vi "Serial_CommModule.vi"(8 "error in (no error)":errorcluster) -> (0 "error out":errorcluster)   [LabVIEW 2021]
uses:
  QueueEnum.ctl
  TCPCommModuleData.ctl
  TCPQueueData.ctl
  TCPModuleState.ctl
  ModelQueueCluster.ctl
  ToModelSourceEnum.ctl
  FromTCPCluster.ctl
  ToModelFromTCPMessage.ctl
  FormControllerToMOdelCluster.ctl
  ToModelFromControllerEnum.ctl
  ToSerialCommand.ctl
  ToSerialCTL.ctl
  <vilib>/Instr/_visa.llb/VISA Open Access Mode.ctl
  <vilib>/Instr/_visa.llb/VISA Configure Serial Port (Instr).vi
panel:
  out "bytes written":i32
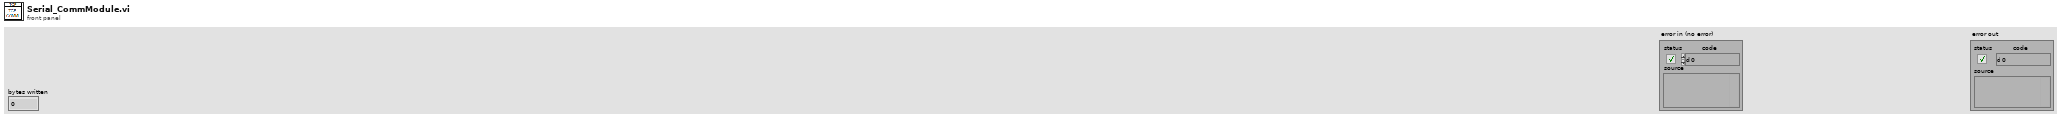
[diagram p1: front panel]
types:
  T1 = typedef "ToSerialCTL.ctl" = enum16{"Init", "Write", "Close", "Read", "Disconnect", "Connect", "Exit", "Error_Handler"}
  T2 = typedef "TCPCommModuleData.ctl" = cluster{"TCP Connection ID":refnum<k5>, "ToTCPModuleQueue":refnum<queue>, "ToModelQueue":refnum<queue>, "Timeout count":u32, "Connected OK?":bool, "ToSerialQueue":refnum<queue>, "VISA resource name":refnum<visa-resource-name>}
  T3 = typedef "QueueEnum.ctl" = enum16{"Obtain Queue", "Get Queue Ref", "Flush Queue", "Release Queue"}
  T4 = enum32{"Invalid", "Standard", "Closed", "Hidden", "Minimized", "Maximized"}
  T5 = typedef "ToSerialCommand.ctl" = cluster{"Command":T1, "VISA resource name":refnum<visa-resource-name>, "Data":string}
  T6 = typedef "ModelQueueCluster.ctl" = cluster{"Source":T7, "FromCommunication":T8, "FromControllerCluster":T10}
  T7 = typedef "ToModelSourceEnum.ctl" = enum16{"COM", "TCP", "Controller"}
  T8 = typedef "FromTCPCluster.ctl" = cluster{"Message":T9, "Data":string, "StatusOK?":bool}
  T9 = typedef "ToModelFromTCPMessage.ctl" = enum16{"Exit", "DataWritten", "DataReceived", "Timeout", "UnableToConnect", "Disconnected", "Connected"}
  T10 = typedef "FormControllerToMOdelCluster.ctl" = cluster{"Command":T11, "IP Address":string, "Remote Port":u16, "Data":string, "TCP/COM":bool, "VISA resource name":refnum<visa-resource-name>}
  T11 = typedef "ToModelFromControllerEnum.ctl" = enum16{"StopLogging", "StartLogging", "SlideChange", "SendMessage", "Exit", "Disconnect", "Connect"}
  T12 = typedef "VISA Open Access Mode.ctl" = u32
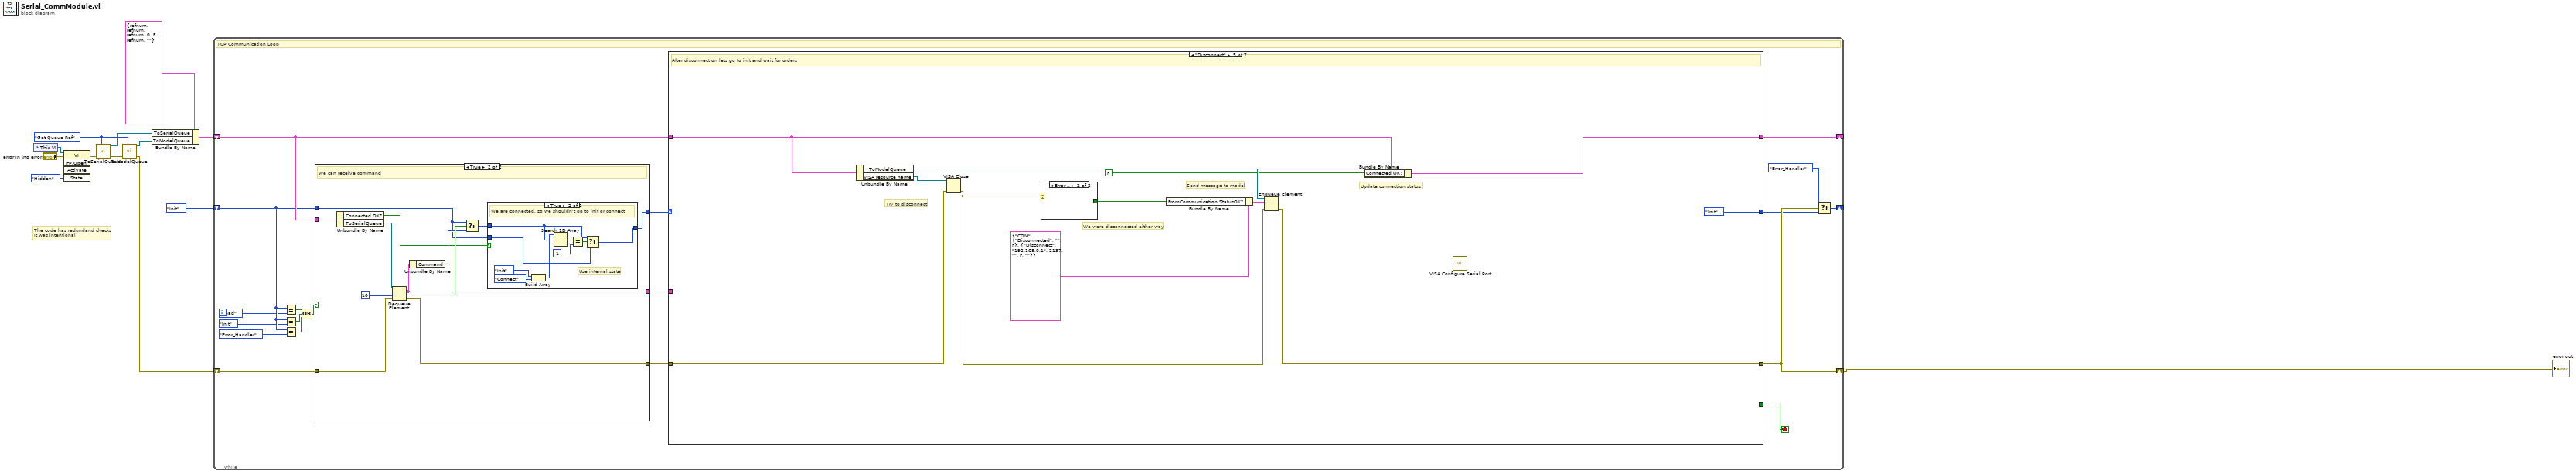
[diagram p0: block diagram]
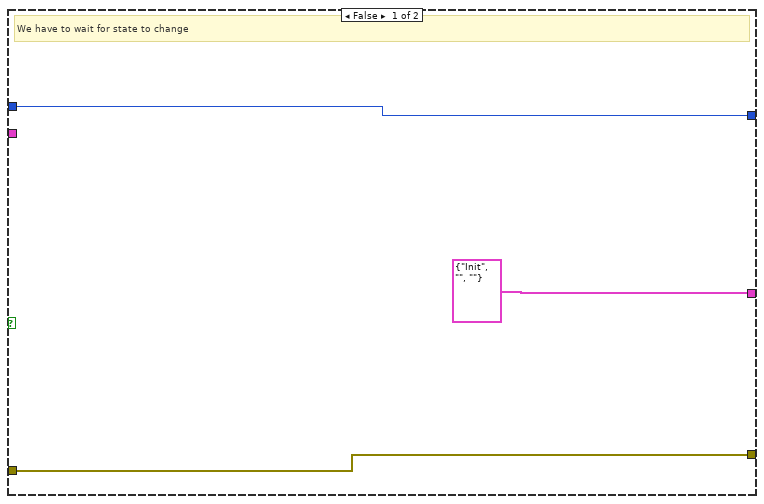
[diagram p2: hidden frame]
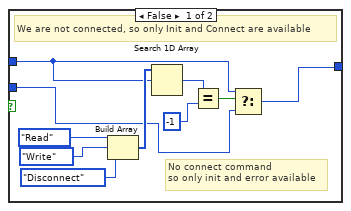
[diagram p3: hidden frame]
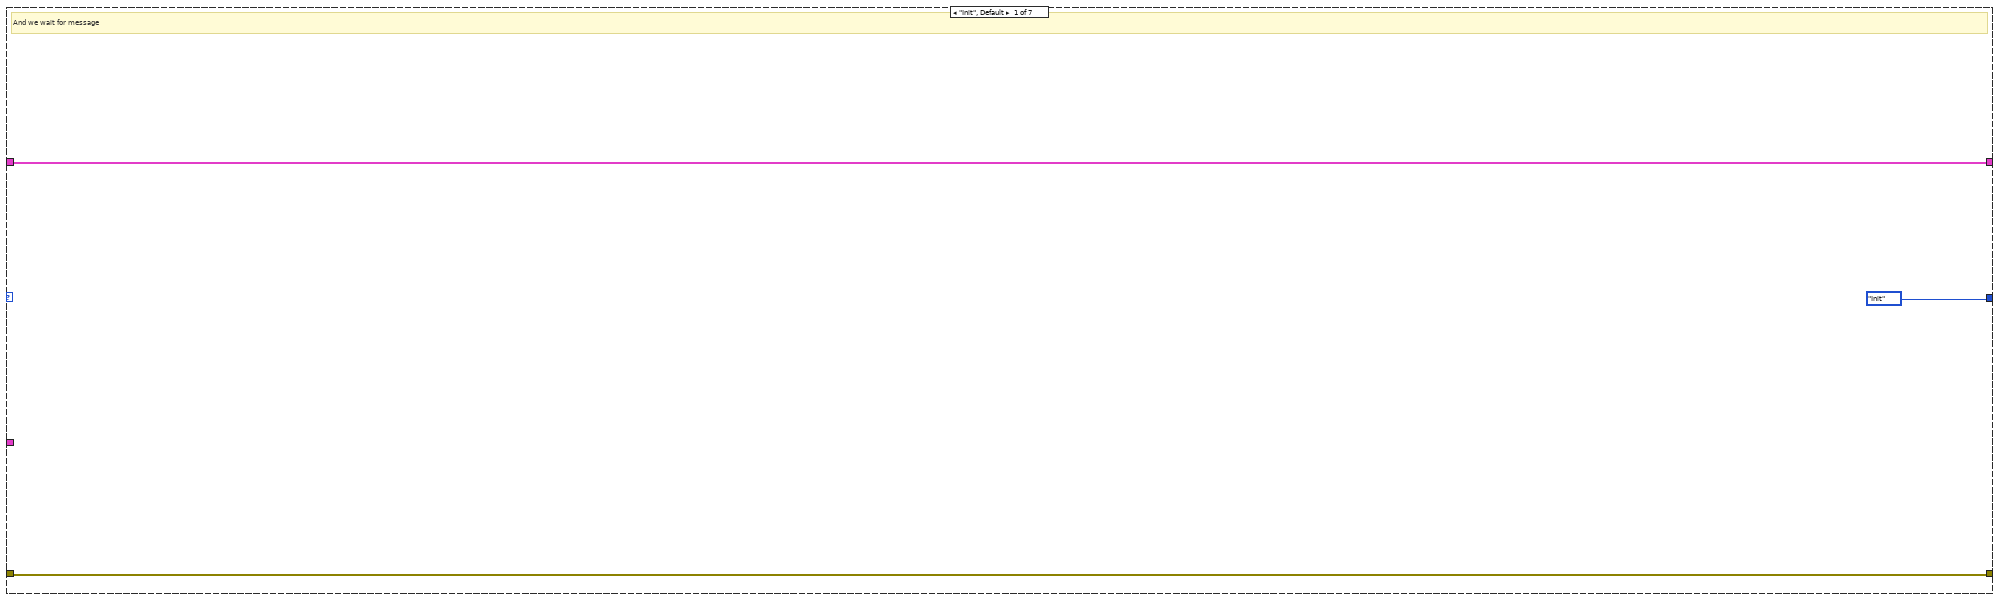
[diagram p4: hidden frame]
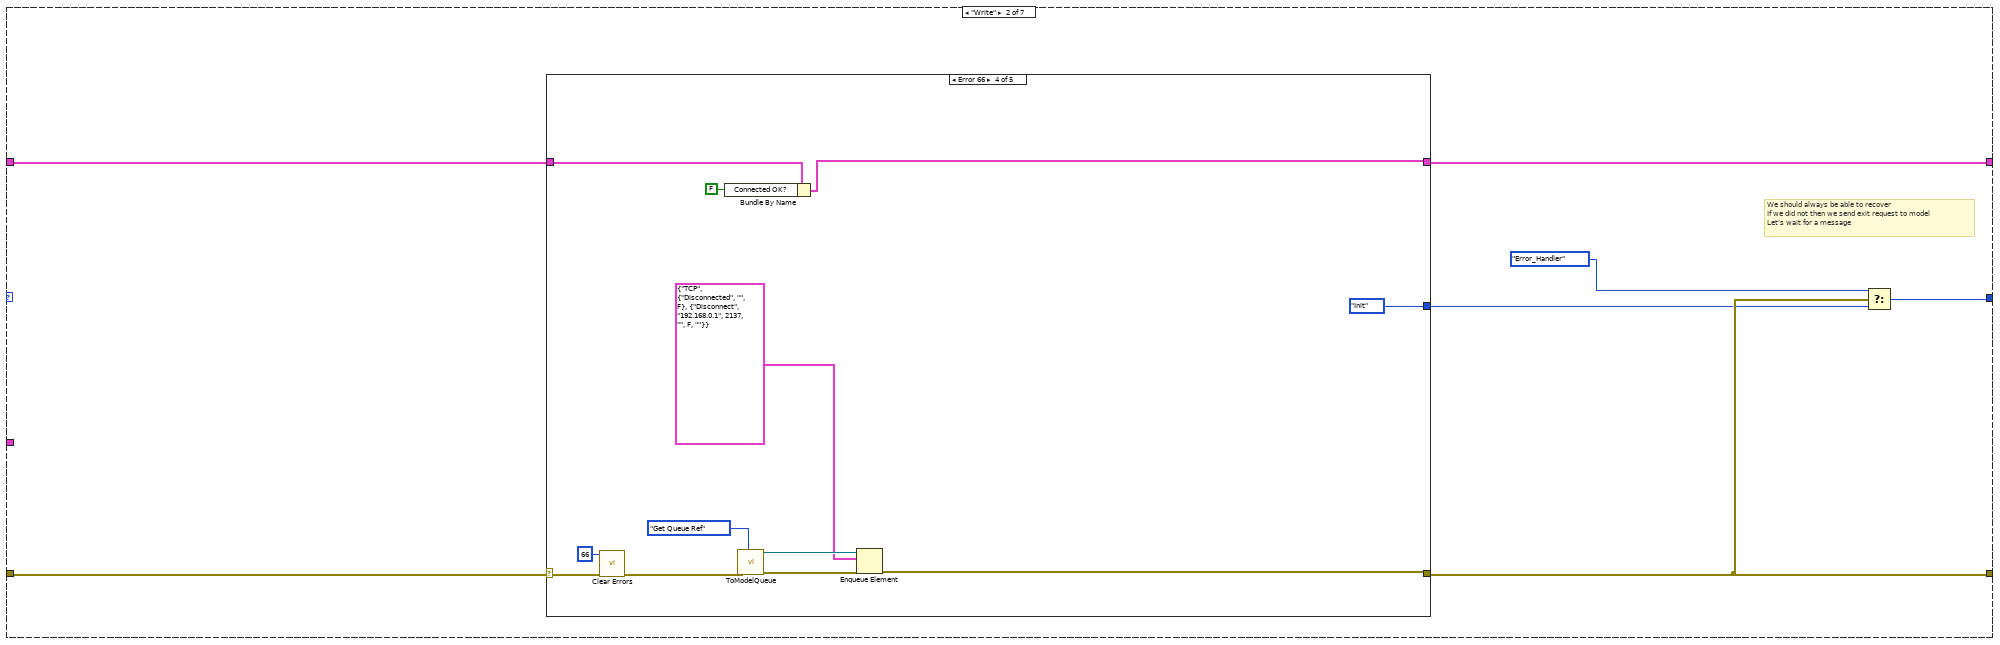
[diagram p5: hidden frame]
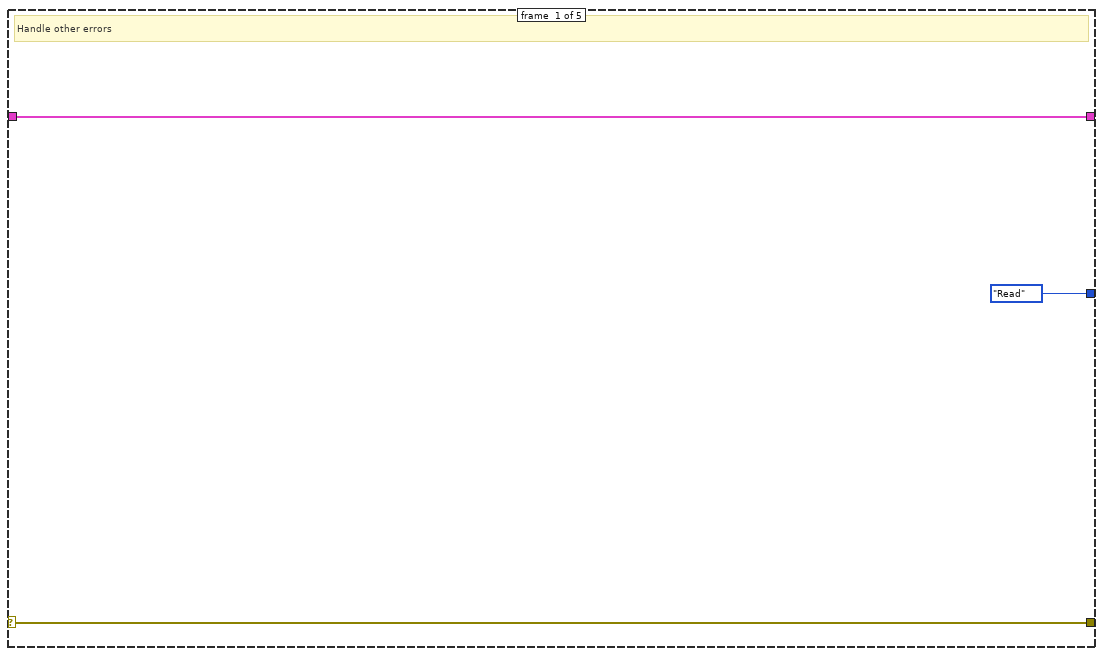
[diagram p6: hidden frame]
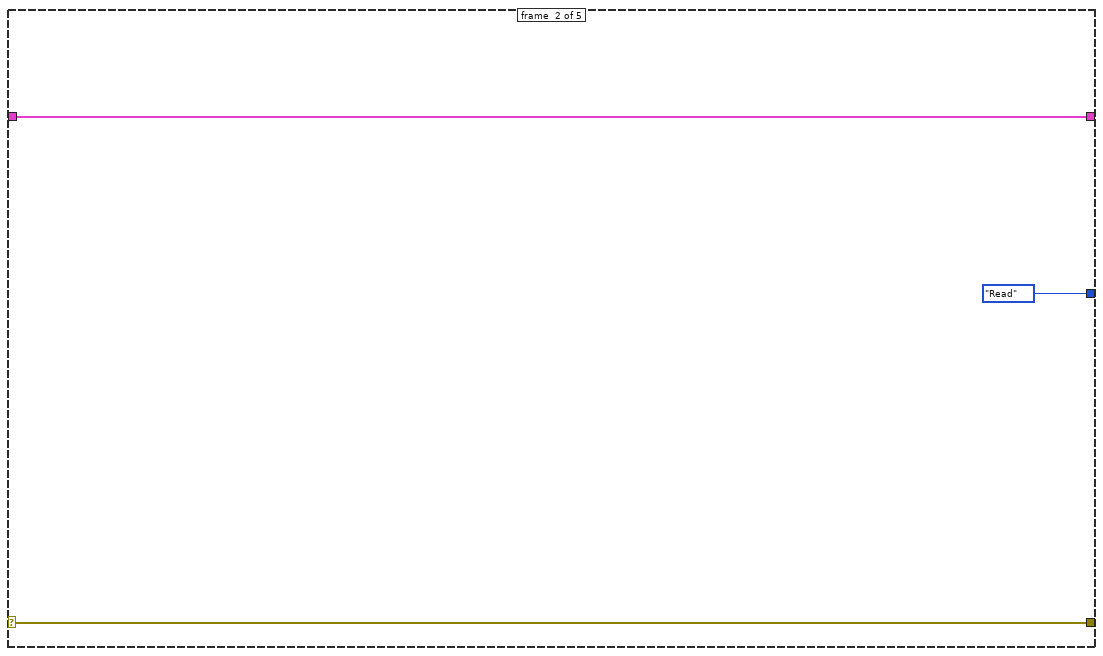
[diagram p7: hidden frame]
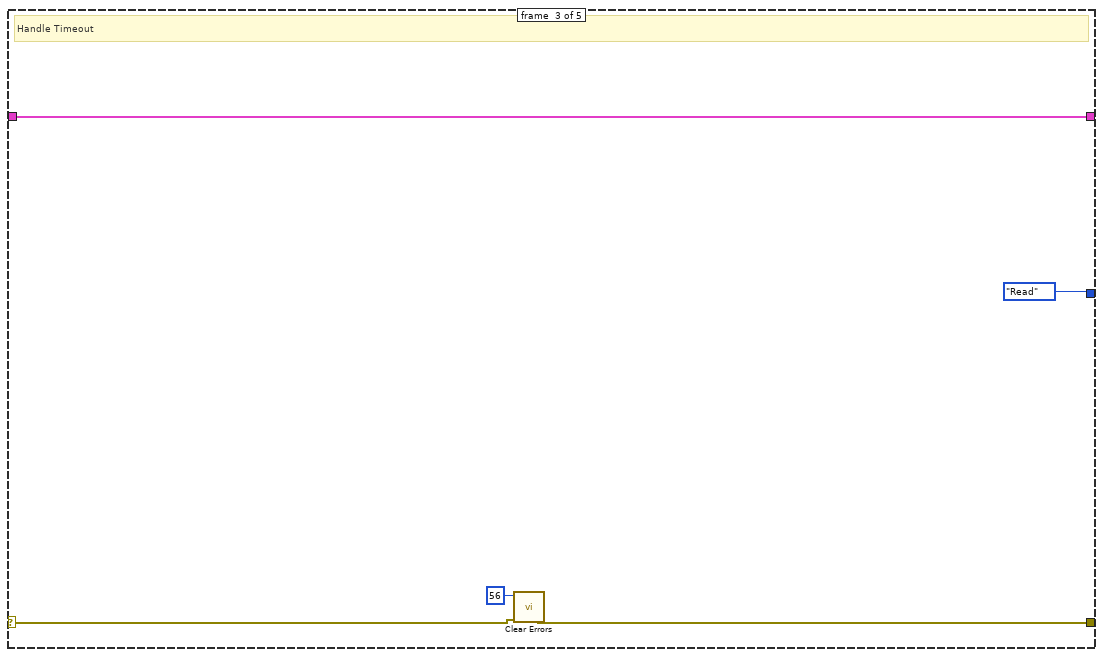
[diagram p8: hidden frame]
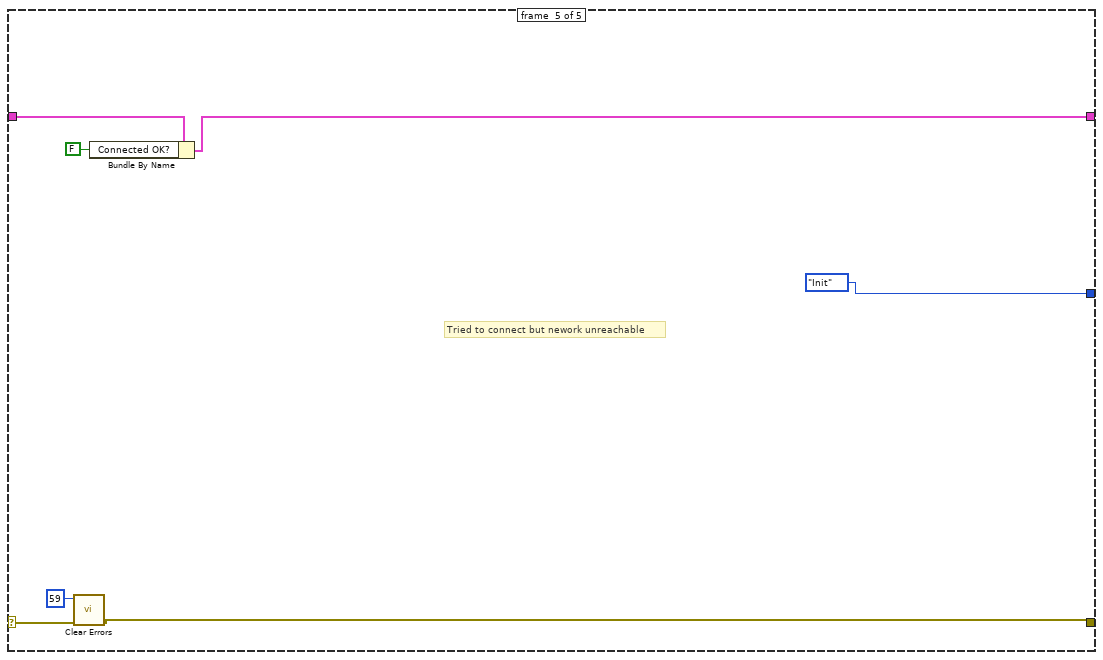
[diagram p9: hidden frame]
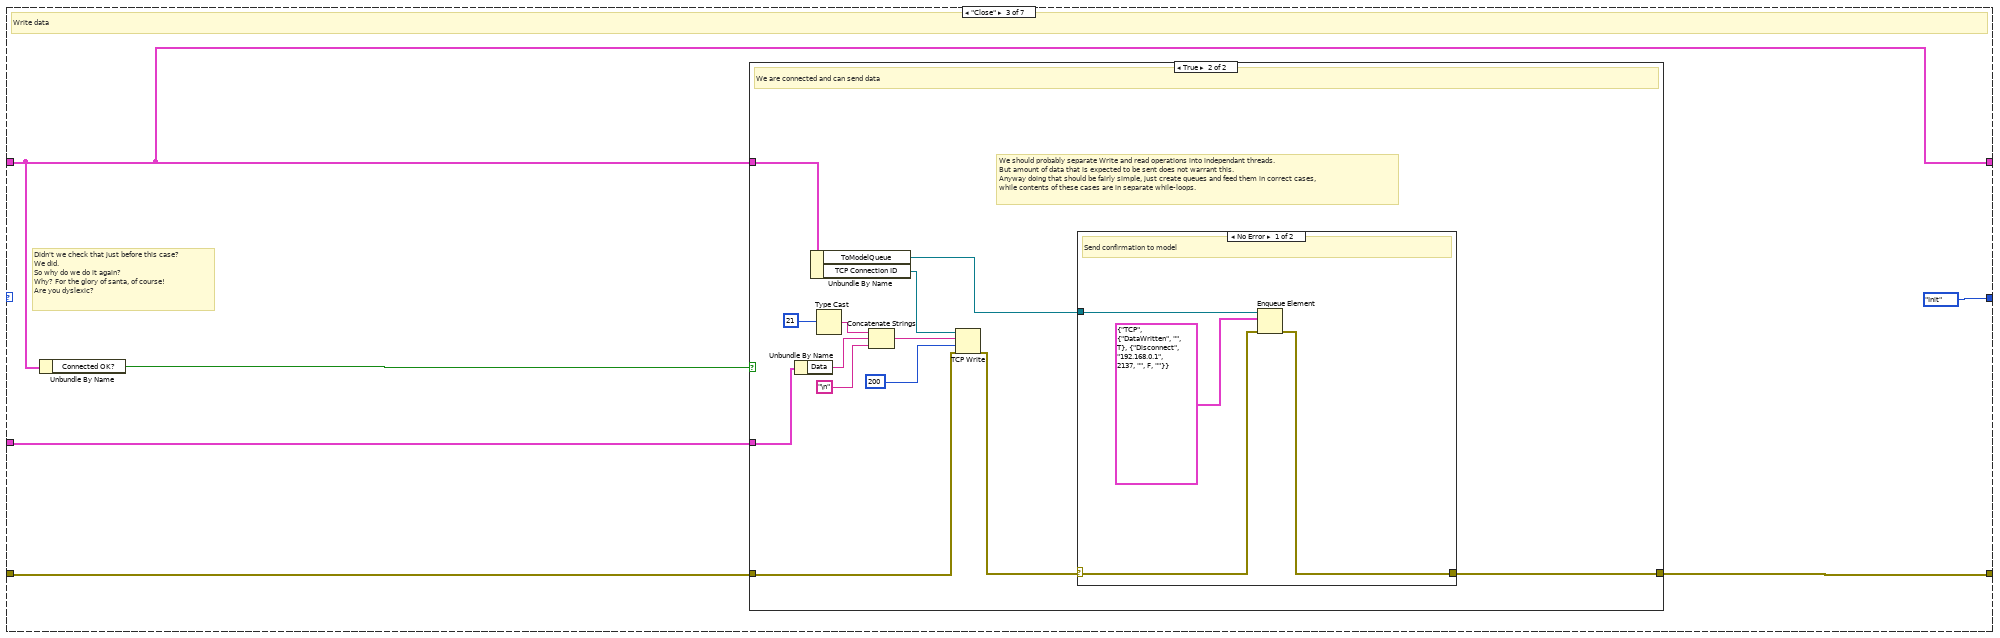
[diagram p10: hidden frame]
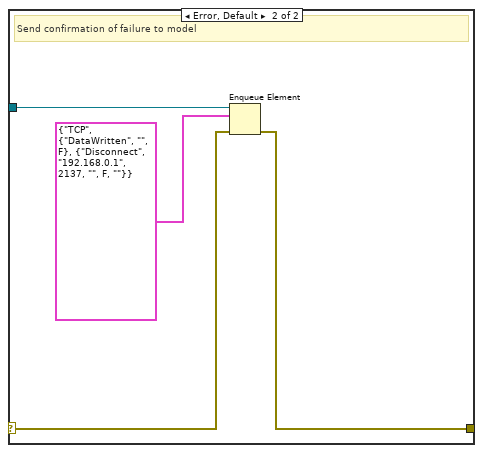
[diagram p12: hidden frame]
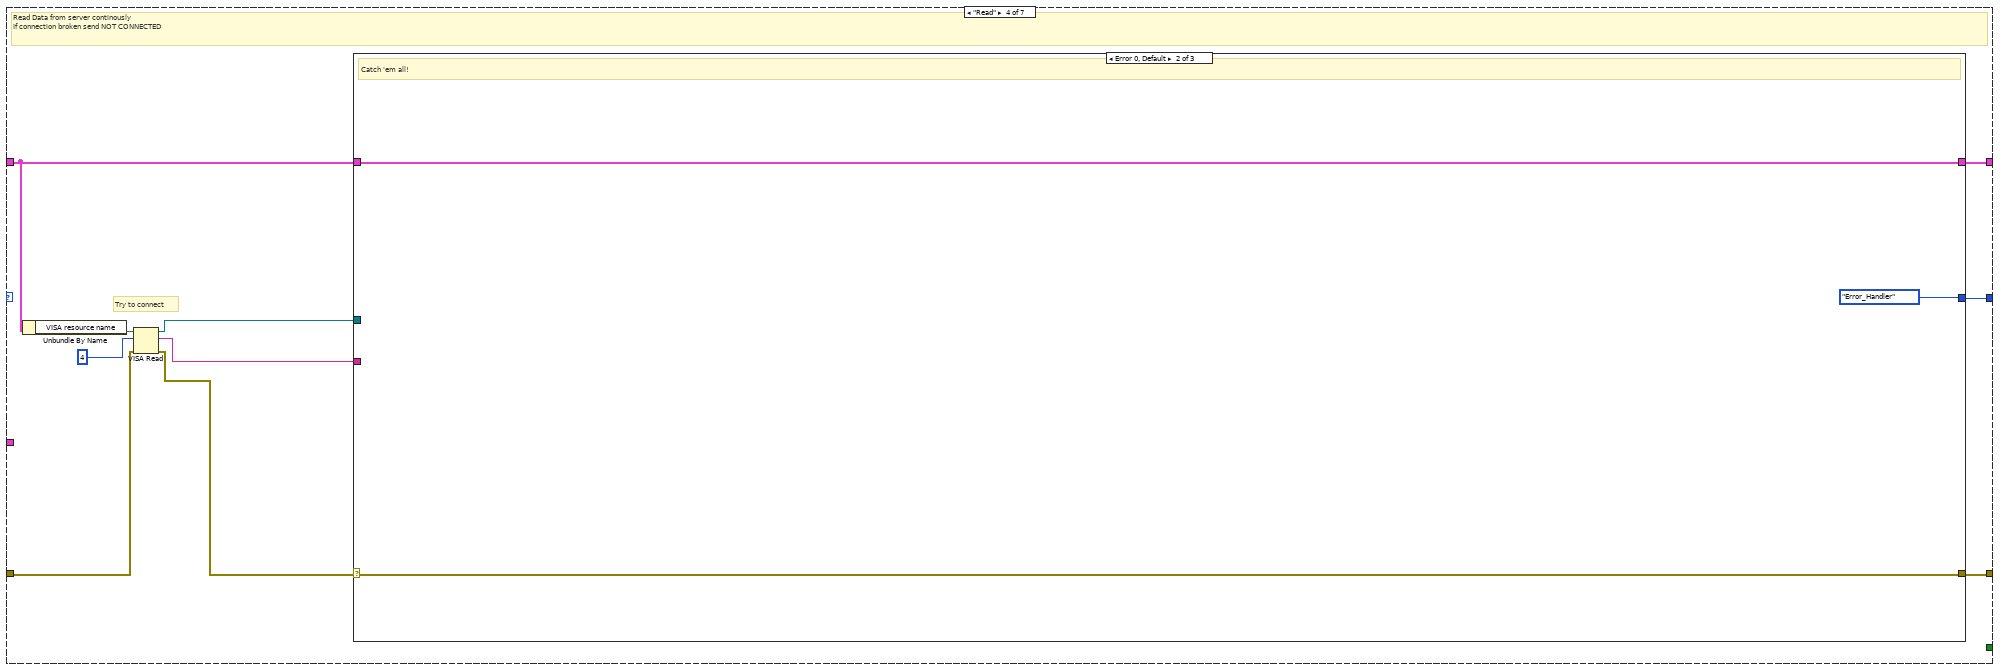
[diagram p13: hidden frame]
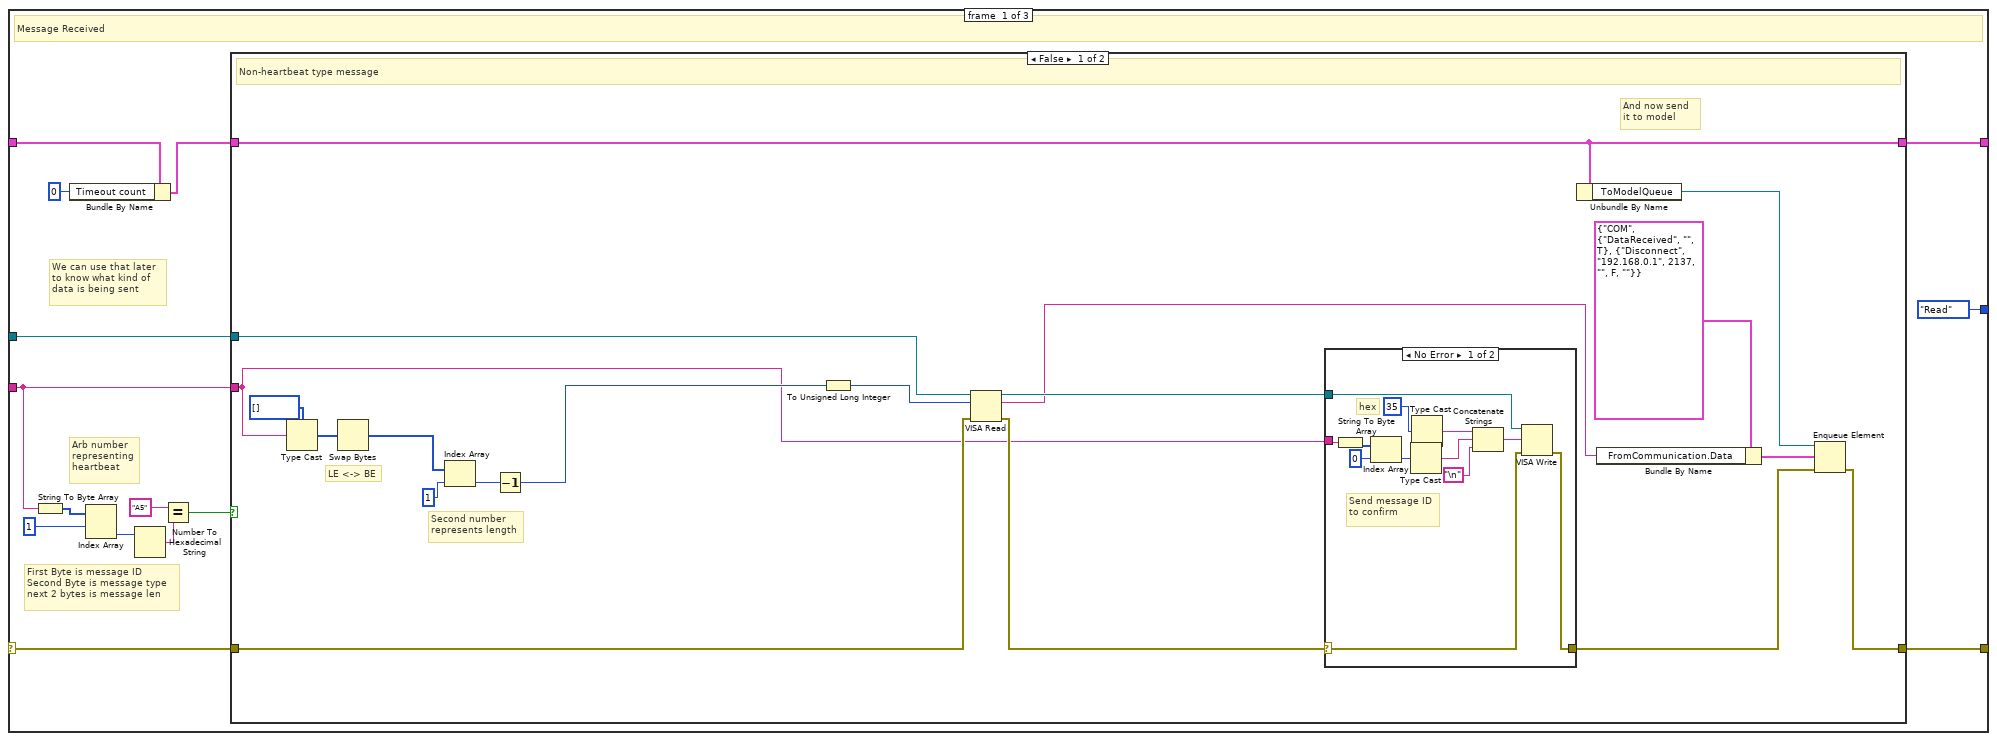
[diagram p14: hidden frame]
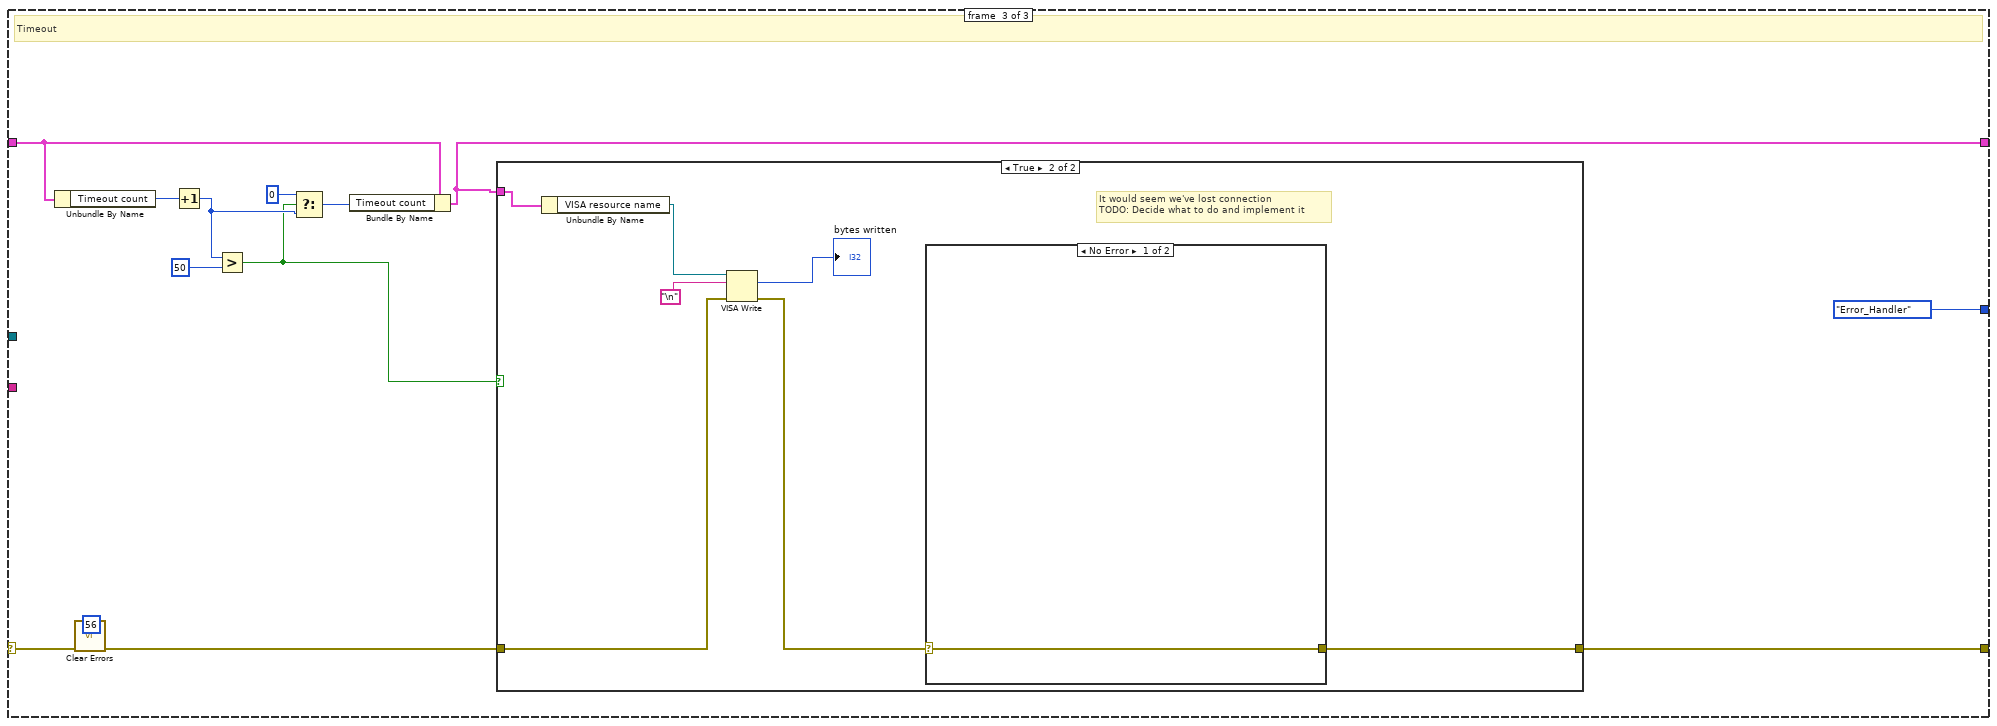
[diagram p17: hidden frame]
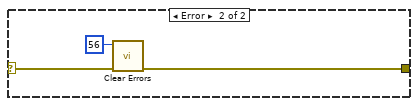
[diagram p19: hidden frame]
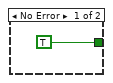
[diagram p20: hidden frame]
diagram:
  w8 = QueueEnum."Get Queue Ref"
  # "The code has redundand checks\nIt was intentional"
  n1 = control-ref of="This VI"() -> (w13:refnum<vi>)
  n2 = invoke class="VI" method="FP.Open"(reference=w13, error in="error in (no error)", "State"=T4."Hidden") -> (error out=w10:errorcluster)  [unwired: 2 in, 4 out]
  n3 = call "ToSerialQueue.vi"("Enum"=w8, "error in (no error)"=w10) -> ("error out"=w9:errorcluster, "queue out"=w6:refnum<queue>)  [unwired: 8 in]
  n4 = call "ToModelQueue.vi"("Enum"=w8, "error in (no error)"=w9) -> ("error out"=w4:errorcluster, "queue out"=w5:refnum<queue>)  [unwired: 8 in]
  n5 = Bundle By Name(cluster=T2 {"TCP Connection ID"=refnum, "ToTCPModuleQueue"=refnum, "ToModelQueue"=refnum, "Timeout count"=0, "Connected OK?"=FALSE, "ToSerialQueue"=refnum, "VISA resource name"=""}, "ToSerialQueue"=w6, "ToModelQueue"=w5) -> (w3:T2)
  n6 = while {
    shift-right: [w25] -> _
    shift-left: ToSerialCTL."Init" ("Command") -> [w18]
    shift-right: [w23] -> _
    shift-left: w3 -> [w27]
    shift-right: [w26] -> w1
    shift-left: w4 -> [w31]
    stop <- w32 stop-if-true
    # "TCP Communication Loop"
    n7 = Equal?(x=w18, y=ToSerialCTL."Read" ("Command")) -> (x = y?=w22:bool)
    n8 = Equal?(x=w18, y=ToSerialCTL."Init" ("Command")) -> (x = y?=w21:bool)
    n9 = Equal?(x=w18, y=ToSerialCTL."Error_Handler" ("Command")) -> (x = y?=w19:bool)
    n10 = Compound Arithmetic op=OR(w22, w21, w19) -> (w20:bool)
    n11 = case shown="True" w20 {
      tunnel: w31 -> [w35 w47]
      tunnel: [w34 w37] -> w30
      tunnel: [w35 w44] -> w29
      tunnel: [T5 {"Command"=enum."Init", "VISA resource name"="", "Data"=""} w42] -> w28
      tunnel: w27 -> [_ w41]
      tunnel: w18 -> [w34 w36]
      frame False {
        # "We have to wait for state to change"
      }
      frame True {
        # "We can receive command"
        n12 = Unbundle By Name(w41) -> ("Connected OK?"=w40:bool, "ToSerialQueue"=w46:refnum<queue>)
        n13 = Dequeue Element(queue=w46, timeout in ms (-1)=10, error in (no error)=w47) -> (element=w42:T5, timed out?=w45:bool, error out=w44:errorcluster)  [unwired: 1 out]
        n14 = Unbundle By Name(w42) -> ("Command"=w39:T1)
        n15 = Select(t=w36, s=w45, f=w39) -> (s? t:f=w38:T1)
        n16 = case shown="True" w40 {
          tunnel: w38 -> [w53 w62]
          tunnel: [w52 w60] -> w37
          tunnel: w36 -> [w51 w61]
          frame False {
            # "No connect command \nso only init and error available"
            # "We are not connected, so only Init and Connect are available"
            n17 = Build Array(ToSerialCTL."Read" ("Command"), ToSerialCTL."Write" ("Command"), ToSerialCTL."Disconnect" ("Command")) -> (w57:T1[])
            n18 = Search 1D Array(1D array=w57, element=w53) -> (index of element=w56:i32)  [unwired: 1 in]
            n19 = Equal?(x=w56, y=-1) -> (x = y?=w54:bool)
            n20 = Select(t=w53, s=w54, f=w51) -> (s? t:f=w52:T1)
          }
          frame True {
            # "Use internal state"
            # "We are connected, so we shouldn't go to init or connect"
            n21 = Build Array(ToSerialCTL."Init" ("Command"), ToSerialCTL."Connect" ("Command")) -> (w66:T1[])
            n22 = Search 1D Array(1D array=w66, element=w62) -> (index of element=w65:i32)  [unwired: 1 in]
            n23 = Equal?(x=w65, y=-1) -> (x = y?=w63:bool)
            n24 = Select(t=w62, s=w63, f=w61) -> (s? t:f=w60:T1)
          }
        }
      }
    }
    n25 = case shown="\"Disconnect\"" w30 {
      tunnel: [_ _ _ _ _ _ TRUE] -> w32
      tunnel: w29 -> [w69 w76 w112 w139 w224 w244 w257]
      tunnel: w28 -> [_ _ w110 _ _ w243 _]
      tunnel: w27 -> [w68 w72 w109 w141 w228 w238 w259]
      tunnel: [w69 w75 w108 w144 w229 w236 w256] -> w26
      tunnel: [ToSerialCTL."Init" ("Command") w74 ToSerialCTL."Init" ("Command") w143 ToSerialCTL."Init" ("Command") ToSerialCTL."Read" ("Command") ToSerialCTL."Exit" ("Command")] -> w24
      tunnel: [w68 w71 w109 w142 w227 w237 w259] -> w23
      frame "Init", Default {
        # "And we wait for message"
      }
      frame "Write" {
        # "We should always be able to recover\nIf we did not then we send exit request to model\nLet's wait for a message"
        n26 = case shown="Error 66" w76 {
          selector: w76 -> [w79 w82 w85 w99 w106]
          tunnel: [w79 w82 w86 w92 w104] -> w75
          tunnel: [ToSerialCTL."Read" ("Command") ToSerialCTL."Read" ("Command") ToSerialCTL."Read" ("Command") ToSerialCTL."Init" ("Command") ToSerialCTL."Init" ("Command")] -> w73
          tunnel: w72 -> [w78 w81 w84 w91 w103]
          tunnel: [w78 w81 w84 w89 w101] -> w71
          frame #0 {
            # "Handle other errors"
          }
          frame #1 {
          }
          frame #2 {
            # "Handle Timeout"
            n27 = call <vilib>:"Clear Errors.vi"("error in (no error)"=w85, "specific error code to clear (0: all)"=56) -> ("error out"=w86:errorcluster)  [unwired: 4 in, 1 out]
          }
          frame #3 {
            n28 = call <vilib>:"Clear Errors.vi"("error in (no error)"=w99, "specific error code to clear (0: all)"=66) -> ("error out"=w97:errorcluster)  [unwired: 4 in, 1 out]
            n29 = Bundle By Name(cluster=w91, "Connected OK?"=FALSE) -> (w89:T2)
            n30 = call "ToModelQueue.vi"("Enum"=QueueEnum."Get Queue Ref", "error in (no error)"=w97) -> ("error out"=w95:errorcluster, "queue out"=w94:refnum<queue>)  [unwired: 8 in]
            n31 = Enqueue Element(queue=w94, element=T6 {"Source"=enum."TCP", "FromCommunication"={"Message"=enum."Disconnected", "Data"="", "StatusOK?"=FALSE}, "FromControllerCluster"={"Command"=enum."Disconnect", "IP Address"="192.168.0.1", "Remote Port"=2137, "Data"="", "TCP/COM"=FALSE, "VISA resource name"=""}}, error in (no error)=w95) -> (error out=w92:errorcluster)  [unwired: 1 in, 2 out]
          }
          frame #4 {
            # "Tried to connect but nework unreachable"
            n32 = call <vilib>:"Clear Errors.vi"("error in (no error)"=w106, "specific error code to clear (0: all)"=59) -> ("error out"=w104:errorcluster)  [unwired: 4 in, 1 out]
            n33 = Bundle By Name(cluster=w103, "Connected OK?"=FALSE) -> (w101:T2)
          }
        }
        n34 = Select(t=ToSerialCTL."Error_Handler" ("Command"), s=w75, f=w73) -> (s? t:f=w74:T1)
      }
      frame "Close" {
        # "Didn't we check that just before this case?\nWe did.\nSo why do we do it again?\nWhy? For the glory of santa, of course!\nAre you dyslexic?"
        # "Write data"
        n35 = Unbundle By Name(w109) -> ("Connected OK?"=w111:bool)
        n36 = case shown="True" w111 {
          tunnel: w112 -> [w113 w124]
          tunnel: w109 -> [_ w126]
          tunnel: w110 -> [_ w122]
          tunnel: [w113 w120] -> w108
          frame False {
            # "Why are we here? Ignore!"
          }
          frame True {
            # "We should probably separate Write and read operations into independant threads.\nBut amount of data that is expected to be sent does not warrant this.\nAnyway doing that should be fairly simple, just create queues and feed them in correct cases,\nwhile contents of these cases are in separate while-loops."
            # "We are connected and can send data"
            n37 = Unbundle By Name(w122) -> ("Data"=w118:string)
            n38 = Unbundle By Name(w126) -> ("ToModelQueue"=w119:refnum<queue>, "TCP Connection ID"=w125:refnum<k5>)
            n39 = Type Cast(x=u8 21) -> (*(type *) &x=w114:string)  [unwired: 1 in]
            n40 = Concatenate Strings(w114, w118, "\n") -> (w117:string)
            n41 = TCP Write(connection ID=w125, data in=w117, error in (no error)=w124, 9:200 ("timeout ms (25000)")) -> (error out=w121:errorcluster)  [unwired: 2 out]
            n42 = case shown="No Error" w121 {
              selector: w121 -> [w129 w133]
              tunnel: [w128 w132] -> w120
              tunnel: w119 -> [w130 w134]
              frame No Error {
                # "Send confirmation to model"
                n43 = Enqueue Element(queue=w130, element=T6 {"Source"=enum."TCP", "FromCommunication"={"Message"=enum."DataWritten", "Data"="", "StatusOK?"=TRUE}, "FromControllerCluster"={"Command"=enum."Disconnect", "IP Address"="192.168.0.1", "Remote Port"=2137, "Data"="", "TCP/COM"=FALSE, "VISA resource name"=""}}, error in (no error)=w129) -> (error out=w128:errorcluster)  [unwired: 1 in, 2 out]
              }
              frame Error, Default {
                # "Send confirmation of failure to model"
                n44 = Enqueue Element(queue=w134, element=T6 {"Source"=enum."TCP", "FromCommunication"={"Message"=enum."DataWritten", "Data"="", "StatusOK?"=FALSE}, "FromControllerCluster"={"Command"=enum."Disconnect", "IP Address"="192.168.0.1", "Remote Port"=2137, "Data"="", "TCP/COM"=FALSE, "VISA resource name"=""}}, error in (no error)=w133) -> (error out=w132:errorcluster)  [unwired: 1 in, 2 out]
              }
            }
          }
        }
      }
      frame "Read" {
        # "Try to connect"
        # "Read Data from server continously\nIf connection broken send NOT CONNECTED"
        n45 = Unbundle By Name(w141) -> ("VISA resource name"=w140:refnum<visa-resource-name>)
        n46 = VISA Read(VISA resource name=w140, byte count=u32 4, error in (no error)=w139) -> (VISA resource name out=w136:refnum<visa-resource-name>, read buffer=w137:string, error out=w138:errorcluster)  [unwired: 1 out]
        n47 = case shown="Error 0, Default" w138 {
          selector: w138 -> [w150 w196 w209]
          tunnel: w136 -> [w151 _ _]
          tunnel: [w156 w196 w202] -> w144
          tunnel: [ToSerialCTL."Read" ("Command") ToSerialCTL."Error_Handler" ("Command") ToSerialCTL."Error_Handler" ("Command")] -> w143
          tunnel: w141 -> [w154 w195 w206]
          tunnel: [w155 w195 w204] -> w142
          tunnel: w137 -> [w146 _ _]
          frame #0 {
            # "First Byte is message ID\nSecond Byte is message type\nnext 2 bytes is message len"
            # "We can use that later \nto know what kind of\ndata is being sent"
            # "Arb number\nrepresenting\nheartbeat"
            # "Message Received"
            n48 = String To Byte Array(string=w146) -> (unsigned byte array=w149:u8[])
            n49 = Bundle By Name(cluster=w154, "Timeout count"=u32 0) -> (w153:T2)
            n50 = Index Array(array=w149, index #1=1 ("index")) -> (element #2=w147:u8)  [unwired: 1 in, 1 out]
            n51 = Number To Hexadecimal String(2:w147) -> (0:w159:string)  [unwired: 1 in]
            n52 = Equal?(x="A5", y=w159) -> (x = y?=w157:bool)
            n53 = case shown="False" w157 {
              tunnel: w150 -> [w167 w193]
              tunnel: [w175 w193] -> w156
              tunnel: w151 -> [w165 _]
              tunnel: w153 -> [w177 w192]
              tunnel: [w177 w192] -> w155
              tunnel: w146 -> [w161 _]
              frame False {
                # "LE <-> BE"
                # "Second number\nrepresents length"
                # "And now send\nit to model"
                # "Non-heartbeat type message"
                n54 = Type Cast(type=u16[] [], x=w161) -> (*(type *) &x=w171:u16[])
                n55 = Swap Bytes(anything=w171) -> (byte swapped=w170:u16[])
                n56 = Index Array(array=w170, index=1) -> (element=w169:u16)
                n57 = Decrement(x=w169) -> (x-1=w166:u16)
                n58 = To Unsigned Long Integer(number=w166) -> (unsigned 32bit integer=w162:u32)
                n59 = VISA Read(VISA resource name=w165, byte count=w162, error in (no error)=w167) -> (VISA resource name out=w163:refnum<visa-resource-name>, read buffer=w160:string, error out=w164:errorcluster)  [unwired: 1 out]
                n60 = case shown="No Error" w164 {
                  selector: w164 -> [w180 w191]
                  tunnel: w161 -> [w190 _]
                  tunnel: w163 -> [w181 _]
                  tunnel: [w179 w191] -> w168
                  frame No Error {
                    # "hex"
                    # "Send message ID\nto confirm"
                    n61 = String To Byte Array(string=w190) -> (unsigned byte array=w189:u8[])
                    n62 = Index Array(array=w189, index=0) -> (element=w187:u8)
                    n63 = Type Cast(x=w187) -> (*(type *) &x=w186:string)  [unwired: 1 in]
                    n64 = Type Cast(x=u8 35) -> (*(type *) &x=w183:string)  [unwired: 1 in]
                    n65 = Concatenate Strings(w183, w186, "\n") -> (w182:string)
                    n66 = VISA Write(VISA resource name=w181, write buffer=w182, error in (no error)=w180) -> (error out=w179:errorcluster)  [unwired: 2 out]
                  }
                  frame Error {
                    # "Decide how to handle\nmessage not received"
                  }
                }
                n67 = Unbundle By Name(w177) -> ("ToModelQueue"=w176:refnum<queue>)
                n68 = Bundle By Name(cluster=T6 {"Source"=enum."COM", "FromCommunication"={"Message"=enum."DataReceived", "Data"="", "StatusOK?"=TRUE}, "FromControllerCluster"={"Command"=enum."Disconnect", "IP Address"="192.168.0.1", "Remote Port"=2137, "Data"="", "TCP/COM"=FALSE, "VISA resource name"=""}} ("element"), "FromCommunication.Data"=w160) -> (w173:T6)
                n69 = Enqueue Element(queue=w176, element=w173, error in (no error)=w168) -> (error out=w175:errorcluster)  [unwired: 1 in, 2 out]
              }
              frame True {
                # "We can check here if device is alive\nDevice should send periodic heartbeat messages.\nThough in this particular project we expect\ncontinous data flow from ToF sensors so this is redundant.\nBut can be useful in future."
                # "Heartbeat\nContinue"
              }
            }
          }
          frame #1 {
            # "Catch 'em all!"
          }
          frame #2 {
            # "Timeout"
            n70 = Unbundle By Name(w206) -> ("Timeout count"=w207:u32)
            n71 = call <vilib>:"Clear Errors.vi"("error in (no error)"=w209, "specific error code to clear (0: all)"=56) -> ("error out"=w203:errorcluster)  [unwired: 4 in, 1 out]
            n72 = Increment(x=w207) -> (x+1=w200:u32)
            n73 = Greater?(x=w200, y=u32 50) -> (0:w198:bool)
            n74 = Select(t=u32 0, s=w198, f=w200) -> (s? t:f=w201:u32)
            n75 = Bundle By Name(cluster=w206, "Timeout count"=w201) -> (w204:T2)
            n76 = case shown="True" w198 {
              tunnel: w204 -> [_ w217]
              tunnel: w203 -> [w210 w213]
              tunnel: [w210 w216] -> w202
              frame False {
              }
              frame True {
                # "It would seem we've lost connection\nTODO: Decide what to do and implement it"
                n77 = Unbundle By Name(w217) -> ("VISA resource name"=w215:refnum<visa-resource-name>)
                n78 = VISA Write(VISA resource name=w215, write buffer="\n", error in (no error)=w213) -> (return count=→"bytes written":u32, error out=w212:errorcluster)  [unwired: 1 out]
                n79 = case shown="No Error" w212 {
                  selector: w212 -> [w218 w221]
                  tunnel: [w218 w220] -> w216
                  frame No Error {
                  }
                  frame Error {
                    n80 = call <vilib>:"Clear Errors.vi"("error in (no error)"=w221, "specific error code to clear (0: all)"=56) -> ("error out"=w220:errorcluster)  [unwired: 4 in, 1 out]
                  }
                }
              }
            }
          }
        }
      }
      frame "Disconnect" {
        # "Update connection status"
        # "Send message to model"
        # "Try to disconnect"
        # "We were disconnected either way"
        # "After disconnection lets go to init and wait for orders"
        n81 = Unbundle By Name(w228) -> ("ToModelQueue"=w233:refnum<queue>, "VISA resource name"=w223:refnum<visa-resource-name>)
        n82 = VISA Close(VISA resource name=w223, error in (no error)=w224) -> (error out=w222:errorcluster)
        n83 = case shown="Error .." w222 {
          tunnel: [TRUE _] -> w231
          frame No Error {
          }
          frame Error {
          }
        }
        n84 = Bundle By Name(cluster=T6 {"Source"=enum."COM", "FromCommunication"={"Message"=enum."Disconnected", "Data"="", "StatusOK?"=FALSE}, "FromControllerCluster"={"Command"=enum."Disconnect", "IP Address"="192.168.0.1", "Remote Port"=2137, "Data"="", "TCP/COM"=FALSE, "VISA resource name"=""}} ("element"), "FromCommunication.StatusOK?"=w231) -> (w230:T6)
        n85 = Enqueue Element(queue=w233, element=w230, error in (no error)=w222) -> (error out=w229:errorcluster)  [unwired: 1 in, 2 out]
        n86 = Bundle By Name(cluster=w228, "Connected OK?"=FALSE) -> (w227:T2)
      }
      frame "Connect" {
        w241 = T12 0 items=["VISA Defaults"=0, "Exclusive Lock"=1, "Load Configured Settings"=4] ("Access Mode")
        # "Connect to server"
        n87 = Unbundle By Name(w243) -> ("VISA resource name"=w242:refnum<visa-resource-name>)
        n88 = VISA Open(timeout (0)=u32 10 ("VISA Open timeout (0)"), access mode=w241, error in (no error)=w244, VISA resource name=w242) -> (error out=w239:errorcluster)  [unwired: 1 in, 1 out]
        n89 = case shown="Error .." w239 {
          selector: w239 -> [w248 w253]
          tunnel: w238 -> [w249 w252]
          tunnel: [w250 w252] -> w237
          tunnel: [w245 w253] -> w236
          frame No Error {
            n90 = Unbundle By Name(w249) -> ("ToModelQueue"=w247:refnum<queue>)
            n91 = Bundle By Name(cluster=w249, "Connected OK?"=TRUE) -> (w250:T2)
            n92 = Enqueue Element(queue=w247, element=T6 {"Source"=enum."COM", "FromCommunication"={"Message"=enum."Connected", "Data"="", "StatusOK?"=TRUE}, "FromControllerCluster"={"Command"=enum."Disconnect", "IP Address"="192.168.0.1", "Remote Port"=2137, "Data"="", "TCP/COM"=FALSE, "VISA resource name"=""}}, error in (no error)=w248) -> (error out=w245:errorcluster)  [unwired: 1 in, 2 out]
          }
          frame Error {
          }
        }
      }
      frame "Exit" {
        # "Exit"
        n93 = Unbundle By Name(w259) -> ("ToModelQueue"=w258:refnum<queue>)
        n94 = Enqueue Element(queue=w258, element=T6 {"Source"=enum."COM", "FromCommunication"={"Message"=enum."Exit", "Data"="", "StatusOK?"=TRUE}, "FromControllerCluster"={"Command"=enum."Disconnect", "IP Address"="192.168.0.1", "Remote Port"=2137, "Data"="", "TCP/COM"=FALSE, "VISA resource name"=""}}, error in (no error)=w257) -> (error out=w256:errorcluster)  [unwired: 1 in, 2 out]
      }
    }
    n95 = Select(t=ToSerialCTL."Error_Handler" ("Command"), s=w26, f=w24) -> (s? t:f=w25:T1)
  }
  "error out" <- w1
  n96 = call-poly "VISA Configure Serial Port"() -> ()  [unwired: 14 in, 2 out]
